vi "Query Marker.vi"(8 "error in (no error)":errorcluster, 10 "Marker Number (1)":i32=1, 11 "VISA resource name":refnum<visa-resource-name>) -> (0 "error out":errorcluster, 1 "Marker Amplitude":dbl, 2 "Marker Position":dbl, 3 "VISA resource name out":refnum<visa-resource-name>)   [LabVIEW 2013, in "Template - Spectrum Analyzer.lvlib"]
doc: "Returns the x-position and amplitude of a specified marker."
uses:
  <instrlib>/_Template - Spectrum Analyzer/Template - Spectrum Analyzer.lvlib
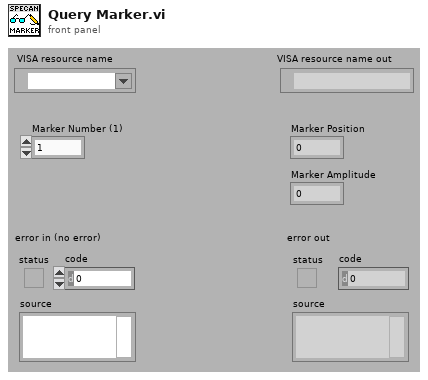
[diagram p1: front panel]
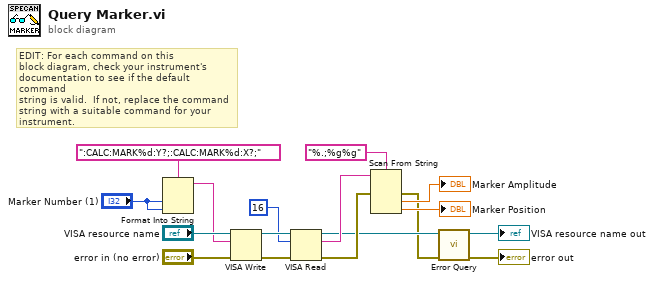
[diagram p0: block diagram]
diagram:
  # "EDIT: For each command on this\nblock diagram, check your instrument's\ndocumentation to see if the default command\nstring is valid.  If not, replace the command\nstring with a suitable command for your\ninstrument."
  n1 = Format Into String(format string=":CALC:MARK%d:Y?;:CALC:MARK%d:X?;", "Marker Number (1)", "Marker Number (1)") -> (resulting string=w11:string)  [unwired: 2 in, 1 out]
  n2 = VISA Write(VISA resource name="VISA resource name", write buffer=w11, error in (no error)="error in (no error)") -> (VISA resource name out=w14:refnum<visa-resource-name>, error out=w15:errorcluster)  [unwired: 1 out]
  n3 = VISA Read(VISA resource name=w14, byte count=u32 16, error in (no error)=w15) -> (VISA resource name out=w4:refnum<visa-resource-name>, read buffer=w7:string, error out=w8:errorcluster)  [unwired: 1 out]
  n4 = Scan From String(format string="%.;%g%g", input string=w7, error in=w8) -> (error out=w3:errorcluster, output 1=→"Marker Amplitude":dbl, output 2=→"Marker Position":dbl)  [unwired: 3 in, 2 out]
  n5 = call <instrlib>:"Error Query.vi"("error in (no error)"=w3, "VISA resource name"=w4) -> ("error out"=→"error out":errorcluster, "VISA resource name out"=→"VISA resource name out":refnum<visa-resource-name>)  [unwired: 6 in, 2 out]
